vi "Cleanup.vi"(8 "error in (no error)":errorcluster, 11 "Terminal in":refnum<class "Terminal.lvclass">) -> (0 "error out":errorcluster)   [LabVIEW 2020, in "Terminal.lvlib" / "Terminal.lvclass"]
uses:
  Terminal.lvclass
  Terminal.lvclass/Terminal.ctl
  <vilib>/IlluminatedG/IG OOPanel/OOPanel/Panel/Panel.lvclass
  TermBuffer/TermBuffer.lvclass
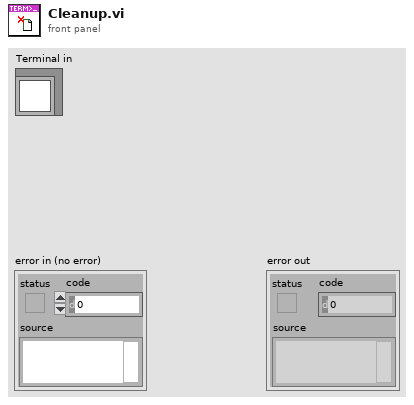
[diagram p1: front panel]
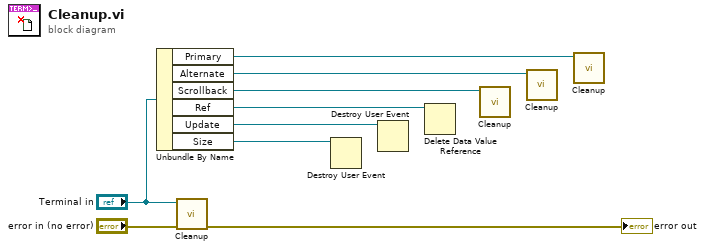
[diagram p0: block diagram]
diagram:
  n1 = Unbundle By Name("Terminal in") -> ("Primary"=w2:refnum<class "TermBuffer.lvclass">, "Alternate"=w3:refnum<class "TermBuffer.lvclass">, "Scrollback"=w4:refnum<class "TermBuffer.lvclass">, "Ref"=w6:refnum<data-value>, "Update"=w5:refnum<user-event>, "Size"=w1:refnum<user-event>)
  n2 = call-parent "Cleanup.vi"("error in (no error)"="error in (no error)", "Panel in"="Terminal in") -> ("error out"=→"error out":errorcluster)  [unwired: 9 in]
  n3 = Destroy User Event(user event=w1) -> ()  [unwired: 1 in, 1 out]
  n4 = Destroy User Event(user event=w5) -> ()  [unwired: 1 in, 1 out]
  n5 = Delete Data Value Reference(data value reference=w6) -> ()  [unwired: 1 in, 2 out]
  n6 = call "Cleanup.vi"("TermBuffer in"=w4) -> ()  [unwired: 10 in, 1 out]
  n7 = call "Cleanup.vi"("TermBuffer in"=w3) -> ()  [unwired: 10 in, 1 out]
  n8 = call "Cleanup.vi"("TermBuffer in"=w2) -> ()  [unwired: 10 in, 1 out]
